vi "Meas Batch Proc QWTB Panel.vi"(8 "error in":errorcluster, 11 "session in":T1={"adc"={"niScope"={"channel cfg"=[], "sessions"=[], "multi cards"=FALSE, "channels"=0, "type"=enum."n/a", "memory [B/chn]"=0, "ext. clock [Hz]"=0.0, "samples count"=0, "use streaming"=FALSE, "proc setup"={"packet size [smpl]"=0, "current timeout [s]"=0.0, "blk2blk timeout [s]"=0.0, "event time"=timestamp(0 s since 1904-01-01), "temp sampl T [s]"=0.0, "data queue"=refnum, "stop notifier"=refnum, "proc ref"=refnum}, "sample width [B]"=0, "ranges [V]"=[], "trigger setup"={"coupling"=1, "level [V]"=0.0, "slope"=0, "mode"=enum."Immediate"}, "fs [Hz]"=0.0, "bitres [bit]"=0}, "3458A"={"channels"=[], "sync unit"={"VISA"="", "type"=enum."Picotest U6200A"}, "awg unit"={"type"=enum."Agilent 331xxA to 332xxA", "VISA"="", "enable 10MHz ref"=FALSE}, "sync mode"=enum."MASTER-SLAVE, MASTER clocked by TIMER", "streaming mode"=FALSE, "idn mode"=enum."Auto", "sampling mode"=enum."DCV", "Ts [s]"=0.0, "sample memory [B]"=0, "proc setup"={"channel id"=0, "packet size [smpl]"=0, "current timeout [s]"=0.0, "blk2blk timeout [s]"=0.0, "event time"=timestamp(0 s since 1904-01-01), "stop notifier"=refnum, "data queues"=[], "proc refs"=[], "bus semaphore"=refnum}, "sample size [B]"=0, "sample count"=0, "aux data"={"channel id"=0, "valid?"=[], "gain [V]"=[], "timestamp [s]"=[], "Ts [s]"=0.0, "abs timestamp"=timestamp(0 s since 1904-01-01), "t [deg C]"=[]}, "ranges [V]"=[], "aperture [s]"=0.0, "LEVEL trigger"={"edge"=enum."POS", "level [V]"=0.0, "coupling"=enum."DC"}, "trigger mode"=enum."AUTO", "measure temp.?"=FALSE, "disp mesages"=[], "shared bus?"=FALSE, "disable display?"=FALSE, "aper mode"=enum."Manual", "aper rules"=[]}, "dsdll"={"dsdll"={"dsdll path"=path "", "dsdll handle"=[], "output devices"=[], "capture devices"=[]}, "channels"=0, "device id"=0, "channel idns"=[], "proc setup"={"packet size [smpl]"=0, "current timeout [s]"=0.0, "blk2blk timeout [s]"=0.0, "event time"=timestamp(0 s since 1904-01-01), "data queue"=refnum, "stop notifier"=refnum, "proc ref"=refnum}, "samples count"=0, "fs [Hz]"=0.0}, "type"=enum."niScope", "channel idn str"=[], "aux instr idn str"=[], "modified?"=FALSE, "simadc"={"channels"=[], "range [V]"=0.0, "Ts step [s]"=0.0, "time [s]"=0.0, "fs [Hz]"=0.0, "count"=0, "smpl offset"=0, "set count"=0, "bit res"=0}, "force rst?"=FALSE, "exit mode"=enum."Immediate reset", "exit dly"=0.0, "exit tmr"=timestamp(0 s since 1904-01-01), "busy?"=FALSE, "accessed?"=FALSE, "QuADC session"={"channel cfg"=[], "sessions"=[], "multi cards"=FALSE, "channels"=0, "type"=enum."n/a", "memory [B/chn]"=0, "ext. clock [Hz]"=0.0, "samples count"=0, "use streaming"=FALSE, "proc setup"={"packet size [smpl]"=0, "current timeout [s]"=0.0, "blk2blk timeout [s]"=0.0, "event time"=timestamp(0 s since 1904-01-01), "temp sampl T [s]"=0.0, "data queue"=refnum, "stop notifier"=refnum, "proc ref"=refnum}, "sample width [B]"=0, "ranges [V]"=[], "trigger setup"={"coupling"=1, "level [V]"=0.0, "slope"=0, "mode"=enum."Immediate"}, "fs [Hz]"=0.0, "bitres [bit]"=0}}, "sequence"=[], "sequence setup"={"group setups"=[], "average cycles"=0, "range mode"=enum."Keep defaults", "fs mode"=enum."Frequency", "rng even"=0.0, "rng odd"=0.0, "folder"=path "", "name base"="", "meas id"=0, "settle [s]"=0.0}, "golpi"=refnum, "processing setup"={"mode"=enum."Raw", "call after avgs?"=FALSE, "calculate?"=FALSE, "raw mode"={"command"="", "result mode"=enum."Display console output (only Octave)", "res variable"=""}, "QWTB"={"QWTB path"=path "", "alg filter path"="", "alg ids"=[], "alg parameters"=[], "parsed parameters"=[], "selected alg id"="", "selected unc mode"=enum."None", "qwtb mcc"=100, "qwtb timeout"=90, "qwtb covg"=95.0, "qwtb ofs"=0, "qwtb lim data"=0, "multicore"={"jobs folder"=path "", "cores"=0, "max jobs"=0, "mode"=enum."Singlecore"}, "unc once?"=FALSE}}, "corrections"={"transducers"={"channels"=[], "last path"=path ""}, "digitizer"={"last path"=path "", "channel paths"=[], "channel idns"=[], "correction name"="", "channel names"=[], "folders to copy"=[], "channel valid"=[], "correction path"=path "", "correction rel path"="", "rel folders to copy"=[]}}, "assist cfg"={"P"=0, "Q"=0, "rel shift"=0.0, "ref freq"=0.0, "min fs"=0.0, "max fs tol"=0.0, "min int"=0.0, "max int"=0.0, "max err"=0.0, "max timeout"=0.0}} {"corrections"."transducers"."channels"."Phase index" min=1 step=1; "adc"."QuADC session"."trigger setup"."level [V]" format="%.2f"; "adc"."QuADC session"."trigger setup"."coupling" items=["AC"=0, "DC"=1, "HF Reject"=3, "LF Reject"=4, "AC Plus HF Reject"=1001]; "adc"."QuADC session"."channel cfg"."Clock fr. (Hz)" min=0.0 format="%#_9p"; "adc"."QuADC session"."channel cfg"."Number of JJ" min=1; "adc"."QuADC session"."channel cfg"."Range [Vpk]" min=0.0; "adc"."QuADC session"."channel cfg"."Channel" min=0; "adc"."3458A"."channels"."Range [Vpk]" min=0.0; "adc"."niScope"."trigger setup"."level [V]" format="%.2f"; "adc"."niScope"."trigger setup"."coupling" items=["AC"=0, "DC"=1, "HF Reject"=3, "LF Reject"=4, "AC Plus HF Reject"=1001]; "adc"."niScope"."channel cfg"."Range [Vpk]" min=0.0; "adc"."niScope"."channel cfg"."Channel" min=0}) -> (0 "error out":errorcluster, 3 "session out":T1={"adc"={"niScope"={"channel cfg"=[], "sessions"=[], "multi cards"=FALSE, "channels"=0, "type"=enum."n/a", "memory [B/chn]"=0, "ext. clock [Hz]"=0.0, "samples count"=0, "use streaming"=FALSE, "proc setup"={"packet size [smpl]"=0, "current timeout [s]"=0.0, "blk2blk timeout [s]"=0.0, "event time"=timestamp(0 s since 1904-01-01), "temp sampl T [s]"=0.0, "data queue"=refnum, "stop notifier"=refnum, "proc ref"=refnum}, "sample width [B]"=0, "ranges [V]"=[], "trigger setup"={"coupling"=1, "level [V]"=0.0, "slope"=0, "mode"=enum."Immediate"}, "fs [Hz]"=0.0, "bitres [bit]"=0}, "3458A"={"channels"=[], "sync unit"={"VISA"="", "type"=enum."Picotest U6200A"}, "awg unit"={"type"=enum."Agilent 331xxA to 332xxA", "VISA"="", "enable 10MHz ref"=FALSE}, "sync mode"=enum."MASTER-SLAVE, MASTER clocked by TIMER", "streaming mode"=FALSE, "idn mode"=enum."Auto", "sampling mode"=enum."DCV", "Ts [s]"=0.0, "sample memory [B]"=0, "proc setup"={"channel id"=0, "packet size [smpl]"=0, "current timeout [s]"=0.0, "blk2blk timeout [s]"=0.0, "event time"=timestamp(0 s since 1904-01-01), "stop notifier"=refnum, "data queues"=[], "proc refs"=[], "bus semaphore"=refnum}, "sample size [B]"=0, "sample count"=0, "aux data"={"channel id"=0, "valid?"=[], "gain [V]"=[], "timestamp [s]"=[], "Ts [s]"=0.0, "abs timestamp"=timestamp(0 s since 1904-01-01), "t [deg C]"=[]}, "ranges [V]"=[], "aperture [s]"=0.0, "LEVEL trigger"={"edge"=enum."POS", "level [V]"=0.0, "coupling"=enum."DC"}, "trigger mode"=enum."AUTO", "measure temp.?"=FALSE, "disp mesages"=[], "shared bus?"=FALSE, "disable display?"=FALSE, "aper mode"=enum."Manual", "aper rules"=[]}, "dsdll"={"dsdll"={"dsdll path"=path "", "dsdll handle"=[], "output devices"=[], "capture devices"=[]}, "channels"=0, "device id"=0, "channel idns"=[], "proc setup"={"packet size [smpl]"=0, "current timeout [s]"=0.0, "blk2blk timeout [s]"=0.0, "event time"=timestamp(0 s since 1904-01-01), "data queue"=refnum, "stop notifier"=refnum, "proc ref"=refnum}, "samples count"=0, "fs [Hz]"=0.0}, "type"=enum."niScope", "channel idn str"=[], "aux instr idn str"=[], "modified?"=FALSE, "simadc"={"channels"=[], "range [V]"=0.0, "Ts step [s]"=0.0, "time [s]"=0.0, "fs [Hz]"=0.0, "count"=0, "smpl offset"=0, "set count"=0, "bit res"=0}, "force rst?"=FALSE, "exit mode"=enum."Immediate reset", "exit dly"=0.0, "exit tmr"=timestamp(0 s since 1904-01-01), "busy?"=FALSE, "accessed?"=FALSE, "QuADC session"={"channel cfg"=[], "sessions"=[], "multi cards"=FALSE, "channels"=0, "type"=enum."n/a", "memory [B/chn]"=0, "ext. clock [Hz]"=0.0, "samples count"=0, "use streaming"=FALSE, "proc setup"={"packet size [smpl]"=0, "current timeout [s]"=0.0, "blk2blk timeout [s]"=0.0, "event time"=timestamp(0 s since 1904-01-01), "temp sampl T [s]"=0.0, "data queue"=refnum, "stop notifier"=refnum, "proc ref"=refnum}, "sample width [B]"=0, "ranges [V]"=[], "trigger setup"={"coupling"=1, "level [V]"=0.0, "slope"=0, "mode"=enum."Immediate"}, "fs [Hz]"=0.0, "bitres [bit]"=0}}, "sequence"=[], "sequence setup"={"group setups"=[], "average cycles"=0, "range mode"=enum."Keep defaults", "fs mode"=enum."Frequency", "rng even"=0.0, "rng odd"=0.0, "folder"=path "", "name base"="", "meas id"=0, "settle [s]"=0.0}, "golpi"=refnum, "processing setup"={"mode"=enum."Raw", "call after avgs?"=FALSE, "calculate?"=FALSE, "raw mode"={"command"="", "result mode"=enum."Display console output (only Octave)", "res variable"=""}, "QWTB"={"QWTB path"=path "", "alg filter path"="", "alg ids"=[], "alg parameters"=[], "parsed parameters"=[], "selected alg id"="", "selected unc mode"=enum."None", "qwtb mcc"=100, "qwtb timeout"=90, "qwtb covg"=95.0, "qwtb ofs"=0, "qwtb lim data"=0, "multicore"={"jobs folder"=path "", "cores"=0, "max jobs"=0, "mode"=enum."Singlecore"}, "unc once?"=FALSE}}, "corrections"={"transducers"={"channels"=[], "last path"=path ""}, "digitizer"={"last path"=path "", "channel paths"=[], "channel idns"=[], "correction name"="", "channel names"=[], "folders to copy"=[], "channel valid"=[], "correction path"=path "", "correction rel path"="", "rel folders to copy"=[]}}, "assist cfg"={"P"=0, "Q"=0, "rel shift"=0.0, "ref freq"=0.0, "min fs"=0.0, "max fs tol"=0.0, "min int"=0.0, "max int"=0.0, "max err"=0.0, "max timeout"=0.0}} {"corrections"."transducers"."channels"."Phase index" min=1 step=1; "adc"."QuADC session"."trigger setup"."level [V]" format="%.2f"; "adc"."QuADC session"."trigger setup"."coupling" items=["AC"=0, "DC"=1, "HF Reject"=3, "LF Reject"=4, "AC Plus HF Reject"=1001]; "adc"."QuADC session"."channel cfg"."Clock fr. (Hz)" min=0.0 format="%#_9p"; "adc"."QuADC session"."channel cfg"."Number of JJ" min=1; "adc"."QuADC session"."channel cfg"."Range [Vpk]" min=0.0; "adc"."QuADC session"."channel cfg"."Channel" min=0; "adc"."3458A"."channels"."Range [Vpk]" min=0.0; "adc"."niScope"."trigger setup"."level [V]" format="%.2f"; "adc"."niScope"."trigger setup"."coupling" items=["AC"=0, "DC"=1, "HF Reject"=3, "LF Reject"=4, "AC Plus HF Reject"=1001]; "adc"."niScope"."channel cfg"."Range [Vpk]" min=0.0; "adc"."niScope"."channel cfg"."Channel" min=0})   [LabVIEW 2018]
doc: "Main panel for QWTB batch processing."
uses:
  Meas Session.ctl
  adc/ADC Session.ctl
  drivers/niScope/niScope Session.ctl
  drivers/niScope/niScope Virtual Channel Config.ctl
  drivers/niScope/niScope Virtual Channel Mode.ctl
  drivers/niScope/niScope Virtual Channel Input Z.ctl
  drivers/niScope/niScope Virtual Channel Coupling.ctl
  drivers/niScope/niScope Type.ctl
  drivers/niScope/niScope Digitizing Process Options.ctl
  drivers/niScope/niScope Data Packet.ctl
  drivers/niScope/niScope Trigger Setup.ctl
  <instrlib>/niScope/Controls/niScope trigger coupling.ctl
  <instrlib>/niScope/Controls/niScope trigger slope.ctl
  drivers/DMM/3458A Digitizer Session.ctl
  drivers/DMM/3458A Virtual Channel Config.ctl
  drivers/Counter/Counter Session.ctl
  drivers/Counter/Counter Type.ctl
  drivers/AWG/AWG Session.ctl
  drivers/AWG/AWG Type.ctl
  drivers/DMM/3458A Sync Mode.ctl
  drivers/DMM/3458A Idn Mode.ctl
  drivers/DMM/3458A Digitizing Low Levels/Configure/Sampling Mode.ctl
  drivers/DMM/3458A Digitizing Process Options.ctl
  drivers/DMM/3458A Data Packet.ctl
  drivers/DMM/3458A Aux Record Data.ctl
  drivers/DMM/3458A Digitizing Low Levels/Configure/Level Setup.ctl
  drivers/DMM/3458A Digitizing Low Levels/Configure/First Sample Trigger.ctl
  drivers/DMM/3458A Aperture Selection Mode.ctl
  drivers/dsdll/DSDLL Session.ctl
  drivers/dsdll/dsdll source distribution/dsdll_instance.ctl
  drivers/dsdll/dsdll source distribution/dsdll_device_record.ctl
  drivers/dsdll/DSDLL Process Config.ctl
  drivers/dsdll/DSDLL Data Packet.ctl
  adc/ADC Type.ctl
  drivers/simulated_adc/SimAdc Config.ctl
  drivers/simulated_adc/SimAdc Channel Cfg.ctl
  adc/ADC On Close Action.ctl
  drivers/Quatsch_driver/QuADCDriver/QuADC Session.ctl
  drivers/Quatsch_driver/QuADCDriver/QuADC Virtual Channel Config.ctl
  drivers/Quatsch_driver/QuADCDriver/QuADC Virtual Channel Mode.ctl
  drivers/Quatsch_driver/QuADCDriver/QuADC Virtual Channel Input Z.ctl
  drivers/Quatsch_driver/QuADCDriver/QuADC Virtual Channel Coupling.ctl
  drivers/Quatsch_driver/QuADCDriver/QuADC Type.ctl
  drivers/Quatsch_driver/QuADCDriver/QuADC Digitizing Process Options.ctl
  drivers/Quatsch_driver/QuADCDriver/QuADC Data Packet.ctl
  drivers/Quatsch_driver/QuADCDriver/QuADC Trigger Setup.ctl
  Meas Sequence Item.ctl
  Meas Sampling Configuration.ctl
  adc/ADC Trig Config.ctl
  adc/ADC Trig Mode Source.ctl
  adc/ADC Trig Coupling.ctl
  adc/ADC Trig Slope.ctl
  Meas Proc QWTB Algorithm Parameter Data.ctl
  Meas Sequence Configuration.ctl
  Meas Range Mode.ctl
  Meas Sampling Rate Mode.ctl
  octave/golpi/mpc/golpi_session_ref.ctl
  octave/golpi/mpc/golpi_session.ctl
  octave/golpi/GOLPI Library.lvlibp/Public/GOLPI reference Type Def.ctl
  octave/golpi/GOLPI Library.lvlibp/LV Process source distribution/Pipe Handle.ctl
  Meas Process Config.ctl
  Meas Process Mode.ctl
  Meas Process Raw Config.ctl
  Meas Process Raw Result Mode.ctl
  Meas Proc QWTB Setup.ctl
  Meas Proc QWTB Uncertainty Mode.ctl
  Meas Proc QWTB Multicore Setup.ctl
  Meas Proc QWTB Multicore Type.ctl
  Corrections/Corr Setup.ctl
  Corrections/Corr Tranducer Item.ctl
  Corrections/Corr Digitizers.ctl
  Assist/Assist Panel Setup.ctl
  varilib/SGUI Assign References Mode.ctl
  octave/infolib.lvlibp/Private/Get key polymorph parts/GetI64.vi
  octave/infolib.lvlibp/Private/Get matrix polymorph parts/Get 1D String.vi
  <vilib>/Utility/error.llb/Error Cluster From Error Code.vi
  varilib/SGUI Assign Multiple Strings With Tags By Label.vi
  <vilib>/ErrorRing/Error Ring.xnode
  octave/infolib.lvlibp
  varilib/varilib.lvlib
  drivers/niScope/niScope Virtual Digitizer.lvlib
  drivers/DMM/3458A Virtual Digitizer.lvlib
  drivers/Counter/Counter.lvlib
  drivers/AWG/AWG.lvlib
  drivers/DMM/3458A Digitizing Low Levels/3458A Digitizing Low Levels.lvlib
  drivers/dsdll/DSDLL Virtual Digitizer.lvlib
  octave/golpi/GOLPI Library.lvlibp/LV Process source distribution/LV Process library.lvlib
  octave/golpi/GOLPI Library.lvlibp
  octave/golpi/mpc/GOLPI Multi Process.lvlib
  drivers/Quatsch_driver/QuADCDriver/QuADC Virtual Digitizer.lvlib
  drivers/dsdll/dsdll source distribution/dsdll.lvlib
panel:
  in  "path history":path caption="Select measurement session"
  in  "btn stop":bool
  out "rec ids":i32[](array[numeric])
  out "group ids unique":i32[](array[numeric])
  out "status":string caption="Status"
  out "group ids":i32[](array[numeric])
  in  "rec list":i32[](listbox) caption="Records available"
  in  "btn cancel":bool
  in  "btn ok":bool
  in  "grp list":i32[](listbox) caption="Groups available"
  in  "meas path":path caption="Select measurement session"
  in  "btn proc":bool
  # "ADC:"
  # "IP Address"
  # "."
  # "."
  # "."
  # ":"
  # "ADC:"
  # "IP Address"
  # "."
  # "."
  # "."
  # ":"
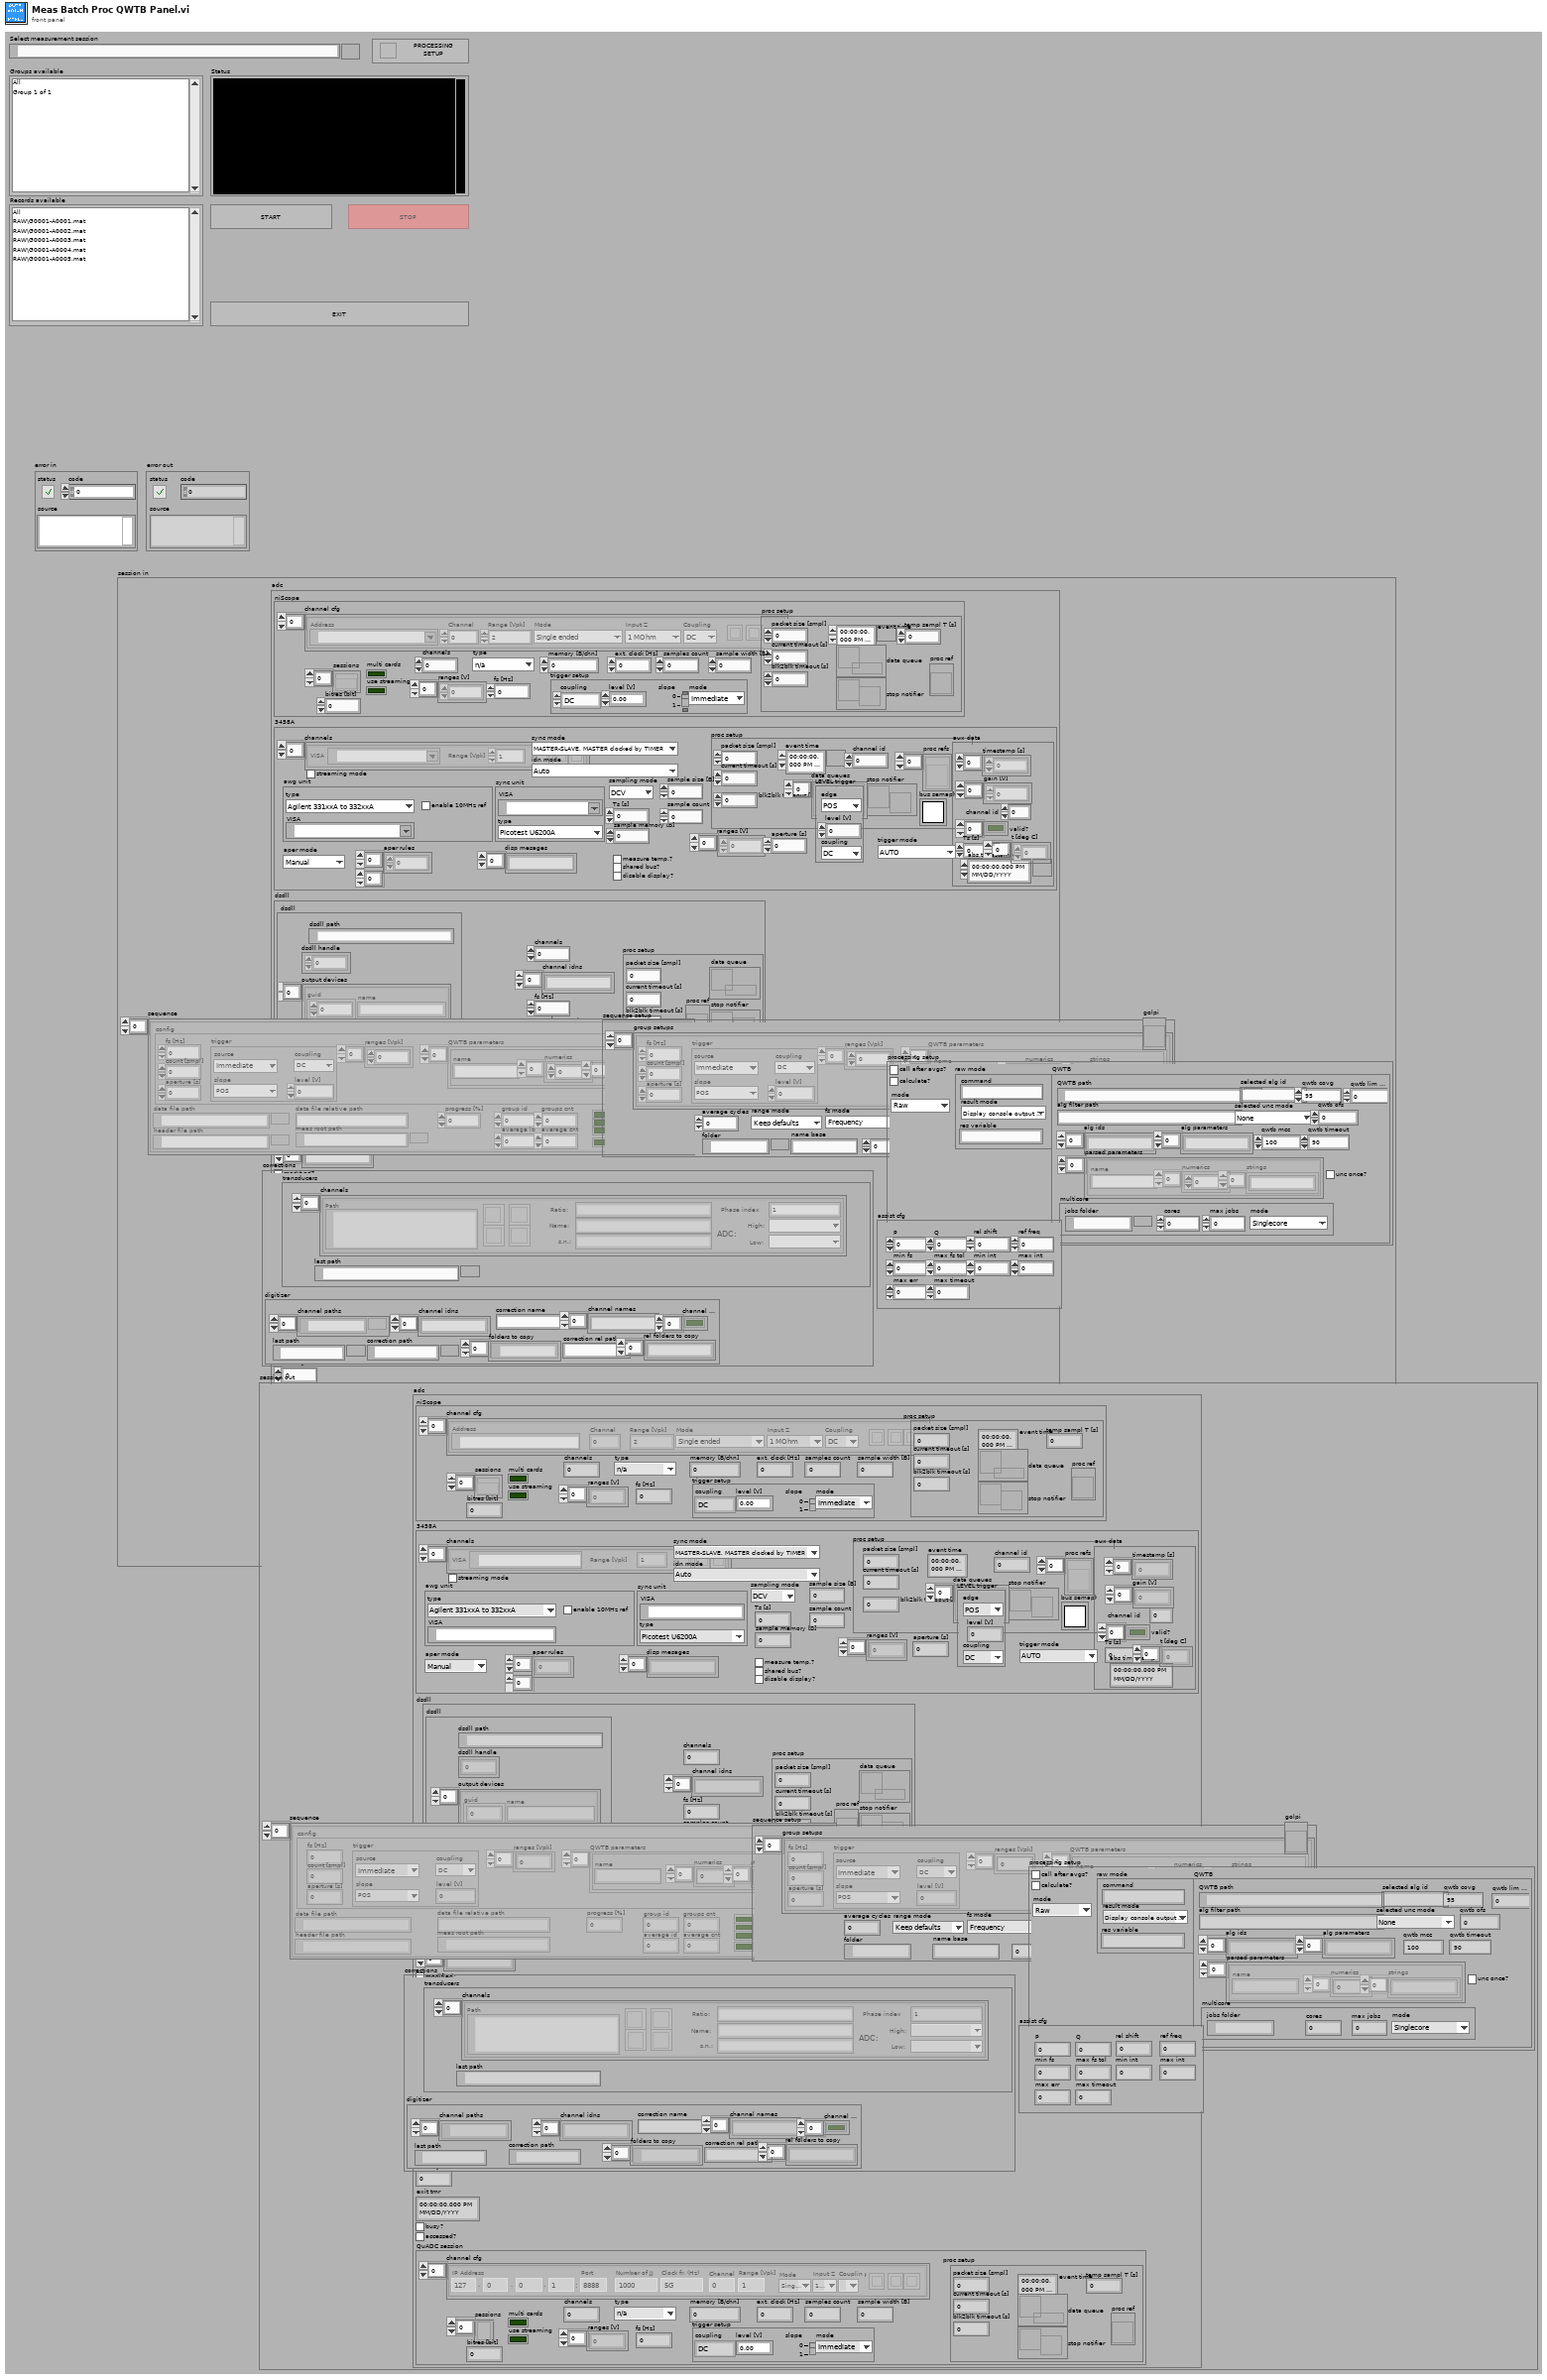
[diagram p1: front panel]
types:
  T1 = typedef "Meas Session.ctl" = cluster{"adc":T2, "sequence":T44[], "sequence setup":T51, "golpi":T54, "processing setup":T55, "corrections":T63, "assist cfg":T66}
  T2 = typedef "ADC Session.ctl" = cluster{"niScope":T3, "3458A":T13, "dsdll":T28, "type":T32, "channel idn str":string[], "aux instr idn str":string[], "modified?":bool, "simadc":T33, "force rst?":bool, "exit mode":T35, "exit dly":dbl, "exit tmr":timestamp, "busy?":bool, "accessed?":bool, "QuADC session":T36}
  T3 = typedef "niScope Virtual Digitizer.lvlib/niScope Session.ctl" = cluster{"channel cfg":T4[], "sessions":refnum<k20>[], "multi cards":bool, "channels":i32, "type":T8, "memory [B/chn]":i32, "ext. clock [Hz]":dbl, "samples count":i64, "use streaming":bool, "proc setup":T9, "sample width [B]":i32, "ranges [V]":dbl[], "trigger setup":T10, "fs [Hz]":dbl, "bitres [bit]":i32}
  T4 = typedef "niScope Virtual Digitizer.lvlib/niScope Virtual Channel Config.ctl" = cluster{"Address":refnum<k15>, "Channel":i32, "Mode":T5, "Input Z":T6, "Coupling":T7, "Range [Vpk]":dbl, "btn clr":bool, "btn up":bool, "btn down":bool}
  T5 = typedef "niScope Virtual Digitizer.lvlib/niScope Virtual Channel Mode.ctl" = enum16{"Single ended", "Unbal. differential", "Differential"}
  T6 = typedef "niScope Virtual Digitizer.lvlib/niScope Virtual Channel Input Z.ctl" = enum16{"1 MOhm", "50 Ohm"}
  T7 = typedef "niScope Virtual Digitizer.lvlib/niScope Virtual Channel Coupling.ctl" = enum16{"AC", "DC", "GND"}
  T8 = typedef "niScope Virtual Digitizer.lvlib/niScope Type.ctl" = enum16{"n/a", "5922"}
  T9 = typedef "niScope Virtual Digitizer.lvlib/niScope Digitizing Process Options.ctl" = cluster{"packet size [smpl]":i64, "current timeout [s]":dbl, "blk2blk timeout [s]":dbl, "event time":timestamp, "temp sampl T [s]":dbl, "data queue":refnum<queue>, "stop notifier":refnum<notifier>, "proc ref":refnum<vi>}
  T10 = typedef "niScope Virtual Digitizer.lvlib/niScope Trigger Setup.ctl" = cluster{"coupling":T11, "level [V]":dbl, "slope":T12, "mode":enum16{"Immediate", "External", "Level"}}
  T11 = typedef "niScope trigger coupling.ctl" = u16
  T12 = typedef "niScope trigger slope.ctl" = i32
  T13 = typedef "3458A Virtual Digitizer.lvlib/3458A Digitizer Session.ctl" = cluster{"channels":T14[], "sync unit":T15, "awg unit":T17, "sync mode":T19, "streaming mode":bool, "idn mode":T20, "sampling mode":T21, "Ts [s]":dbl, "sample memory [B]":i32, "proc setup":T22, "sample size [B]":i32, "sample count":i32, "aux data":T24, "ranges [V]":dbl[], "aperture [s]":dbl, "LEVEL trigger":T25, "trigger mode":T26, "measure temp.?":bool, "disp mesages":string[], "shared bus?":bool, "disable display?":bool, "aper mode":T27, "aper rules":dbl[][]}
  T14 = typedef "3458A Virtual Digitizer.lvlib/3458A Virtual Channel Config.ctl" = cluster{"VISA":refnum<visa-resource-name>, "Range [Vpk]":dbl, "btn clr":bool, "btn up":bool, "btn down":bool}
  T15 = typedef "Counter.lvlib/Counter Session.ctl" = cluster{"VISA":refnum<visa-resource-name>, "type":T16}
  T16 = typedef "Counter.lvlib/Counter Type.ctl" = enum16{"Picotest U6200A", "dummy"}
  T17 = typedef "AWG.lvlib/AWG Session.ctl" = cluster{"type":T18, "VISA":refnum<visa-resource-name>, "enable 10MHz ref":bool}
  T18 = typedef "AWG.lvlib/AWG Type.ctl" = enum16{"Agilent 331xxA to 332xxA", "Agilent 335xxA to 336xxA", "Tektronix AFG3101C", "dummy"}
  T19 = typedef "3458A Virtual Digitizer.lvlib/3458A Sync Mode.ctl" = enum16{"MASTER-SLAVE, MASTER clocked by TIMER", "MASTER-SLAVE, MASTER clocked by AWG", "ALL clocked by AWG", "MASTER-SLAVE, ALL clocked by TIMER", "ALL clocked by AWG with DFLL"}
  T20 = typedef "3458A Virtual Digitizer.lvlib/3458A Idn Mode.ctl" = enum16{"Auto", "Sequential (chn A, chn B, ...)", "From calibration string"}
  T21 = typedef "3458A Virtual Digitizer.lvlib/3458A Digitizing Low Levels.lvlib/Sampling Mode.ctl" = enum16{"DCV", "DSDC", "DSAC"}
  T22 = typedef "3458A Virtual Digitizer.lvlib/3458A Digitizing Process Options.ctl" = cluster{"channel id":i32, "packet size [smpl]":i32, "current timeout [s]":dbl, "blk2blk timeout [s]":dbl, "event time":timestamp, "stop notifier":refnum<notifier>, "data queues":refnum<queue>[], "proc refs":refnum<vi>[], "bus semaphore":T23}
  T23 = typedef "Semaphore RefNum" = refnum<k1>
  T24 = typedef "3458A Virtual Digitizer.lvlib/3458A Aux Record Data.ctl" = cluster{"channel id":i32, "valid?":bool[], "gain [V]":dbl[], "timestamp [s]":dbl[], "Ts [s]":dbl, "abs timestamp":timestamp, "t [deg C]":dbl[]}
  T25 = typedef "3458A Virtual Digitizer.lvlib/3458A Digitizing Low Levels.lvlib/Level Setup.ctl" = cluster{"edge":enum16{"POS", "NEG"}, "level [V]":dbl, "coupling":enum16{"DC", "AC"}}
  T26 = typedef "3458A Virtual Digitizer.lvlib/3458A Digitizing Low Levels.lvlib/First Sample Trigger.ctl" = enum16{"AUTO", "EXT", "SYN", "SGL", "HOLD", "LEVEL"}
  T27 = typedef "3458A Virtual Digitizer.lvlib/3458A Aperture Selection Mode.ctl" = enum16{"Manual", "Maximum", "Table"}
  T28 = typedef "DSDLL Virtual Digitizer.lvlib/DSDLL Session.ctl" = cluster{"dsdll":T29, "channels":i32, "device id":i32, "channel idns":string[], "proc setup":T31, "samples count":i32, "fs [Hz]":dbl}
  T29 = typedef "dsdll.lvlib/dsdll_instance.ctl" = cluster{"dsdll path":path, "dsdll handle":u8[], "output devices":T30[], "capture devices":T30[]}
  T30 = typedef "dsdll.lvlib/dsdll_device_record.ctl" = cluster{"guid":u8[], "name":string}
  T31 = typedef "DSDLL Virtual Digitizer.lvlib/DSDLL Process Config.ctl" = cluster{"packet size [smpl]":i32, "current timeout [s]":dbl, "blk2blk timeout [s]":dbl, "event time":timestamp, "data queue":refnum<queue>, "stop notifier":refnum<notifier>, "proc ref":refnum<vi>}
  T32 = typedef "ADC Type.ctl" = enum16{"niScope", "3458A", "DirectSound DLL", "dummy", "QuADC"}
  T33 = typedef "SimAdc Config.ctl" = cluster{"channels":T34[], "range [V]":dbl, "Ts step [s]":dbl, "time [s]":dbl, "fs [Hz]":dbl, "count":i64, "smpl offset":i64, "set count":i64, "bit res":i32}
  T34 = typedef "SimAdc Channel Cfg.ctl" = cluster{"harmonics":dbl[][], "btn clear":bool, "noise":dbl, "fundamental [Hz]":dbl}
  T35 = typedef "ADC On Close Action.ctl" = enum16{"Immediate reset", "Delayed reset"}
  T36 = typedef "QuADC Virtual Digitizer.lvlib/QuADC Session.ctl" = cluster{"channel cfg":T37[], "sessions":refnum<k5>[], "multi cards":bool, "channels":i32, "type":T41, "memory [B/chn]":i32, "ext. clock [Hz]":dbl, "samples count":i64, "use streaming":bool, "proc setup":T42, "sample width [B]":i32, "ranges [V]":dbl[], "trigger setup":T43, "fs [Hz]":dbl, "bitres [bit]":i32}
  T37 = typedef "QuADC Virtual Digitizer.lvlib/QuADC Virtual Channel Config.ctl" = cluster{"Channel":i32, "Mode":T38, "Input Z":T39, "Coupling":T40, "Range [Vpk]":dbl, "btn clr":bool, "btn up":bool, "btn down":bool, "IP address A":u8, "IP address B":u8, "IP address C":u8, "IP address D":u8, "Port":u16, "Number of JJ":u32, "Clock fr. (Hz)":dbl}
  T38 = typedef "QuADC Virtual Digitizer.lvlib/QuADC Virtual Channel Mode.ctl" = enum16{"Single ended", "Unbal. differential", "Differential"}
  T39 = typedef "QuADC Virtual Digitizer.lvlib/QuADC Virtual Channel Input Z.ctl" = enum16{"1 MOhm", "50 Ohm"}
  T40 = typedef "QuADC Virtual Digitizer.lvlib/QuADC Virtual Channel Coupling.ctl" = enum16{"AC", "DC", "GND"}
  T41 = typedef "QuADC Virtual Digitizer.lvlib/QuADC Type.ctl" = enum16{"n/a", "v1"}
  T42 = typedef "QuADC Virtual Digitizer.lvlib/QuADC Digitizing Process Options.ctl" = cluster{"packet size [smpl]":i64, "current timeout [s]":dbl, "blk2blk timeout [s]":dbl, "event time":timestamp, "temp sampl T [s]":dbl, "data queue":refnum<queue>, "stop notifier":refnum<notifier>, "proc ref":refnum<vi>}
  T43 = typedef "QuADC Virtual Digitizer.lvlib/QuADC Trigger Setup.ctl" = cluster{"coupling":T11, "level [V]":dbl, "slope":T12, "mode":enum16{"Immediate", "External", "Level"}}
  T44 = typedef "Meas Sequence Item.ctl" = cluster{"config":T45, "data file path":path, "header file path":path, "group id":i32, "average id":i32, "group done?":bool, "adc modified?":bool, "source modified?":bool, "progress [%]":dbl, "groups cnt":i32, "average cnt":i32, "data file relative path":string, "meas root path":path, "calculate?":bool}
  T45 = typedef "Meas Sampling Configuration.ctl" = cluster{"fs [Hz]":dbl, "count [smpl]":i64, "aperture [s]":dbl, "trigger":T46, "ranges [Vpk]":dbl[], "QWTB parameters":T50[]}
  T46 = typedef "ADC Trig Config.ctl" = cluster{"source":T47, "level [V]":dbl, "coupling":T48, "slope":T49}
  T47 = typedef "ADC Trig Mode Source.ctl" = enum16{"Immediate", "External", "Level"}
  T48 = typedef "ADC Trig Coupling.ctl" = enum16{"DC", "AC"}
  T49 = typedef "ADC Trig Slope.ctl" = enum16{"POS", "NEG"}
  T50 = typedef "Meas Proc QWTB Algorithm Parameter Data.ctl" = cluster{"name":string, "numerics":dbl[], "strings":string[]}
  T51 = typedef "Meas Sequence Configuration.ctl" = cluster{"group setups":T45[], "average cycles":i32, "range mode":T52, "fs mode":T53, "rng even":dbl, "rng odd":dbl, "folder":path, "name base":string, "meas id":i32, "settle [s]":dbl}
  T52 = typedef "Meas Range Mode.ctl" = enum16{"Keep defaults", "Set All channels", "Set Odd and Even channels"}
  T53 = typedef "Meas Sampling Rate Mode.ctl" = enum16{"Frequency", "Period"}
  T54 = typedef "GOLPI Multi Process.lvlib/golpi_session_ref.ctl" = refnum<vi>
  T55 = typedef "Meas Process Config.ctl" = cluster{"mode":T56, "call after avgs?":bool, "calculate?":bool, "raw mode":T57, "QWTB":T59}
  T56 = typedef "Meas Process Mode.ctl" = enum16{"Raw", "QWTB"}
  T57 = typedef "Meas Process Raw Config.ctl" = cluster{"command":string, "result mode":T58, "res variable":string}
  T58 = typedef "Meas Process Raw Result Mode.ctl" = enum16{"Display console output (only Octave)", "Display string variable", "Display result file %respath%"}
  T59 = typedef "Meas Proc QWTB Setup.ctl" = cluster{"QWTB path":path, "alg filter path":string, "alg ids":string[], "alg parameters":string[], "parsed parameters":T50[], "selected alg id":string, "selected unc mode":T60, "qwtb mcc":i32, "qwtb timeout":i32, "qwtb covg":dbl, "qwtb ofs":i64, "qwtb lim data":i64, "multicore":T61, "unc once?":bool}
  T60 = typedef "Meas Proc QWTB Uncertainty Mode.ctl" = enum16{"None", "GUF", "Monte Carlo"}
  T61 = typedef "Meas Proc QWTB Multicore Setup.ctl" = cluster{"jobs folder":path, "cores":i32, "max jobs":i32, "mode":T62}
  T62 = typedef "Meas Proc QWTB Multicore Type.ctl" = enum16{"Singlecore", "Multicore", "Multistation"}
  T63 = typedef "Corr Setup.ctl" = cluster{"transducers":cluster{"channels":T64[], "last path":path}, "digitizer":T65}
  T64 = typedef "Corr Tranducer Item.ctl" = cluster{"Path":path, "Ratio:":string, "Name:":string, "btn rem":bool, "btn up":bool, "btn down":bool, "s.n.:":string, "btn open":bool, "ratio o/i":dbl, "chn hi":u16, "chn lo":u16, "Phase index":i32}
  T65 = typedef "Corr Digitizers.ctl" = cluster{"last path":path, "channel paths":path[], "channel idns":string[], "correction name":string, "channel names":string[], "folders to copy":path[], "channel valid":bool[], "correction path":path, "correction rel path":string, "rel folders to copy":string[]}
  T66 = typedef "Assist Panel Setup.ctl" = cluster{"P":i32, "Q":i32, "rel shift":dbl, "ref freq":dbl, "min fs":dbl, "max fs tol":dbl, "min int":dbl, "max int":dbl, "max err":dbl, "max timeout":dbl}
  T67 = typedef "varilib.lvlib/SGUI Assign References Mode.ctl" = enum16{"Add to stack", "Overwrite", "Release last", "Release ID"}
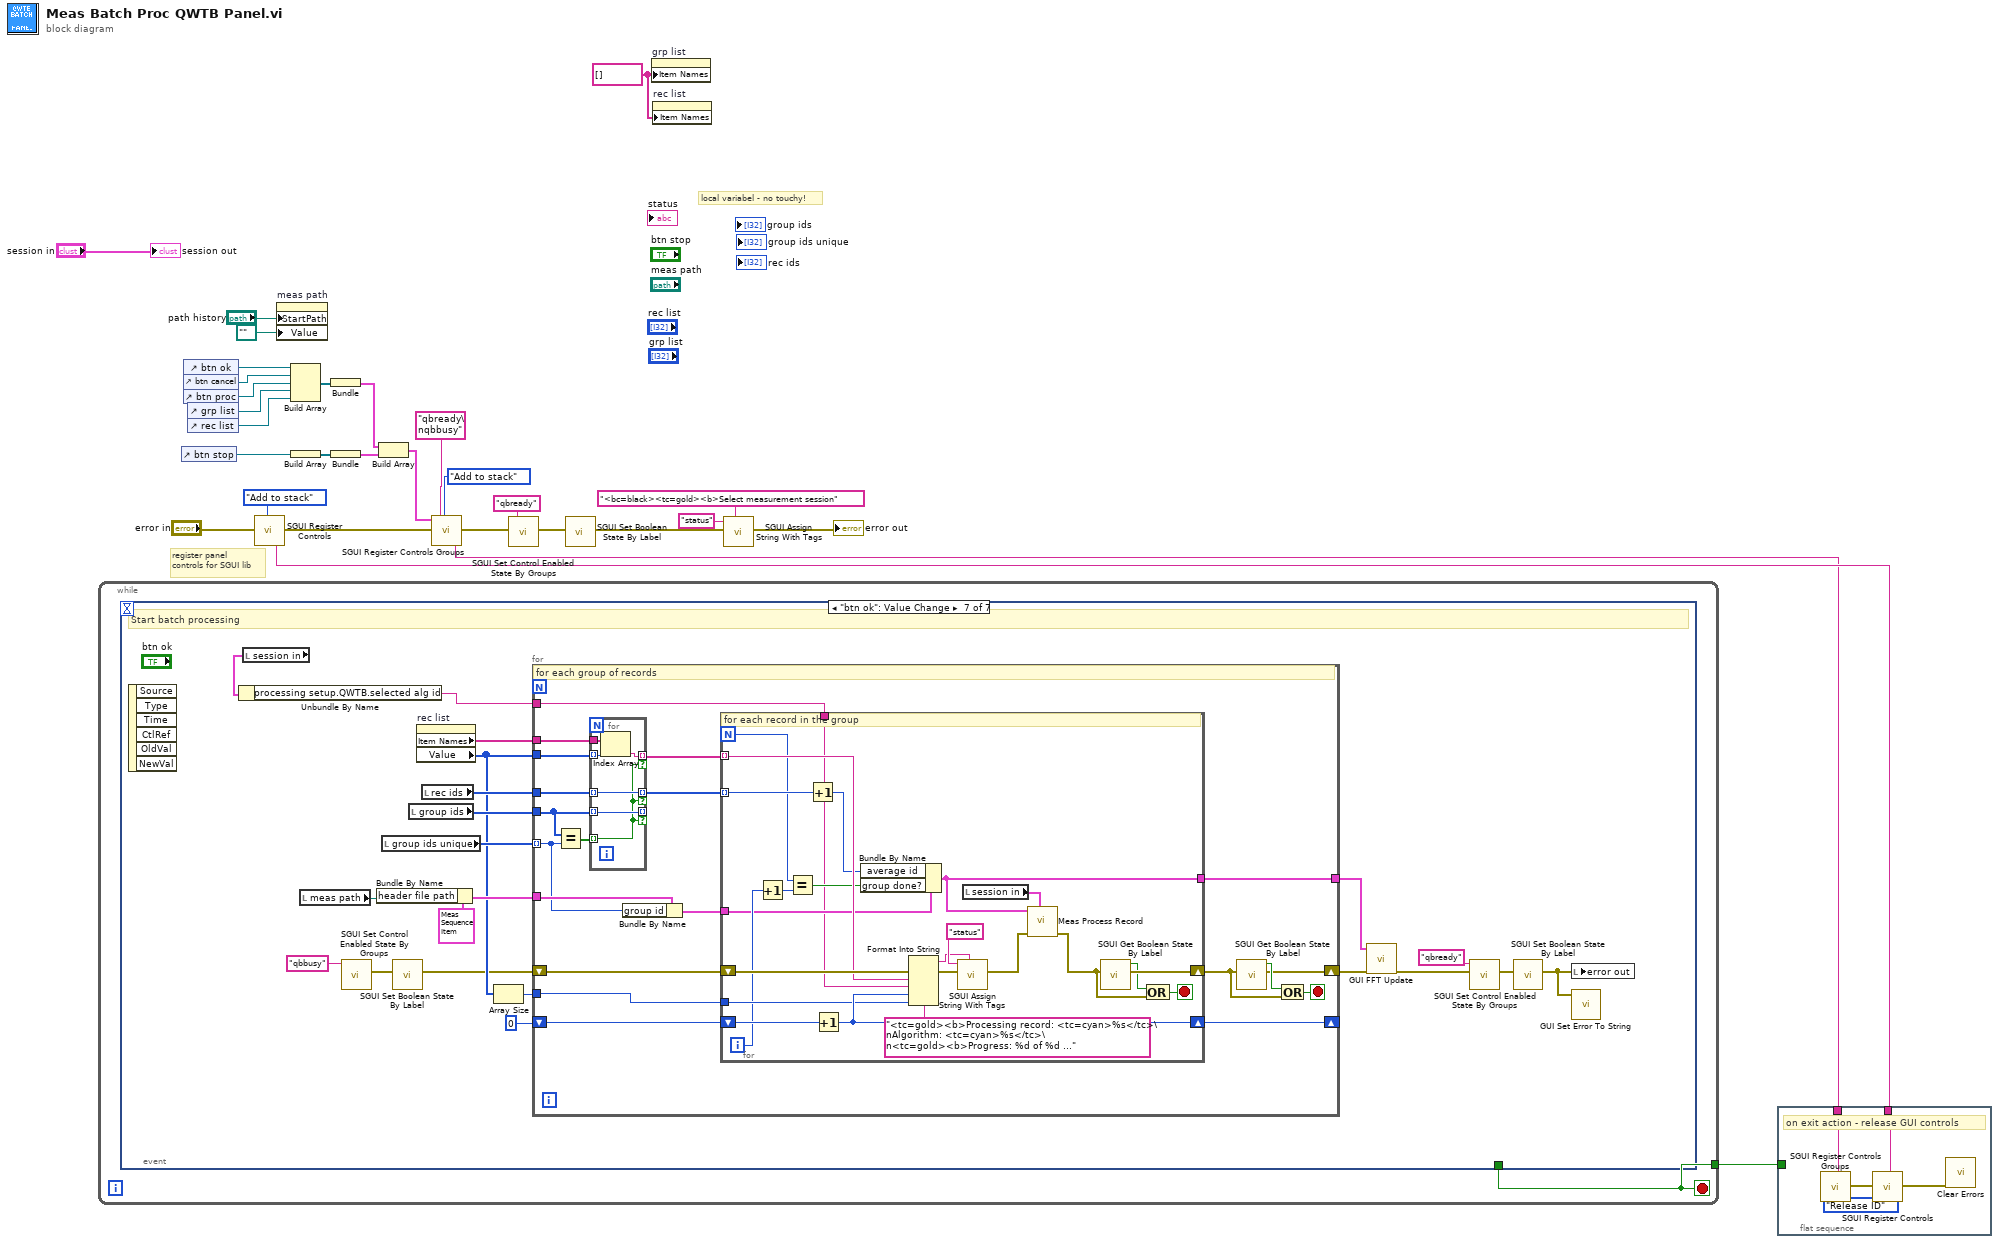
[diagram p0: block diagram]
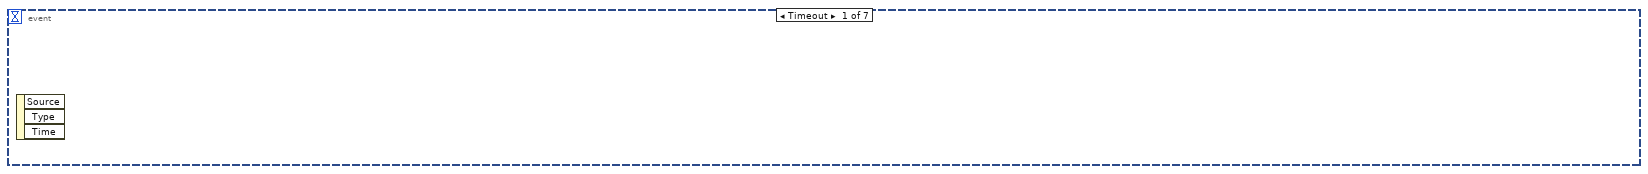
[diagram p2: hidden frame]
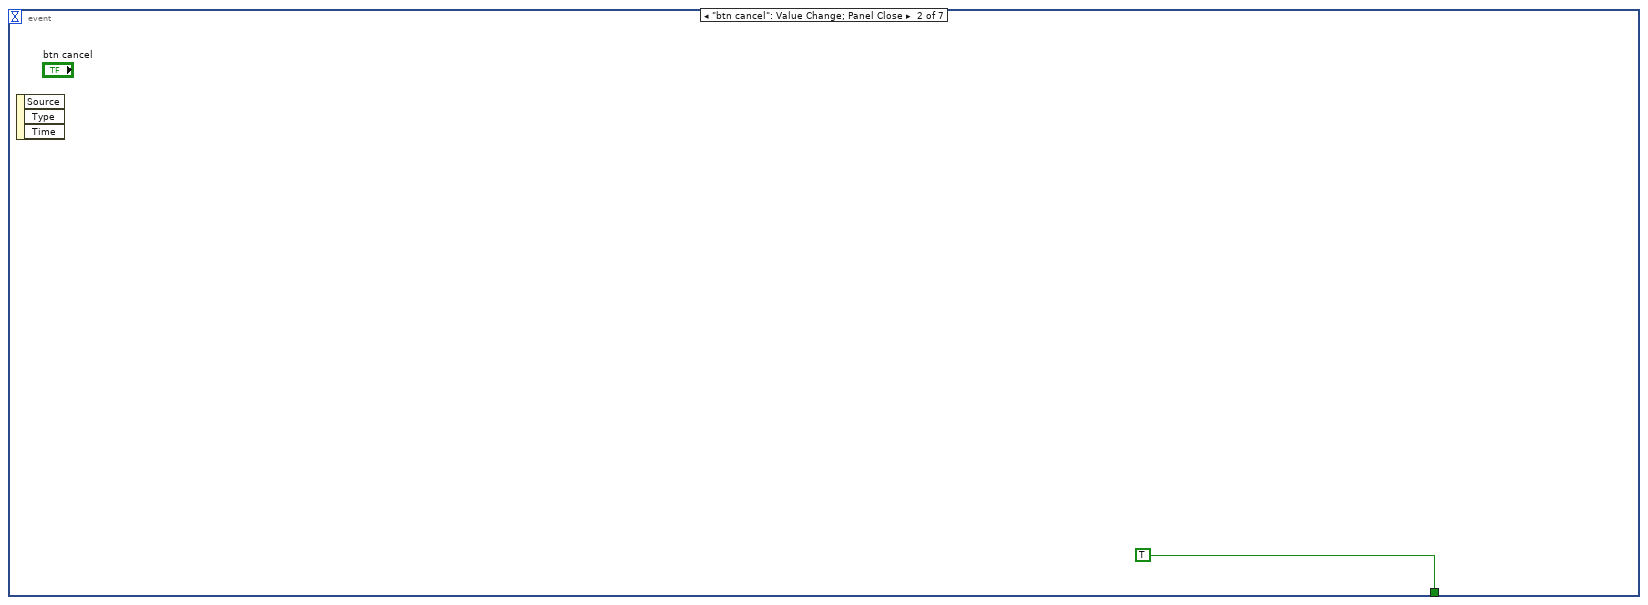
[diagram p3: hidden frame]
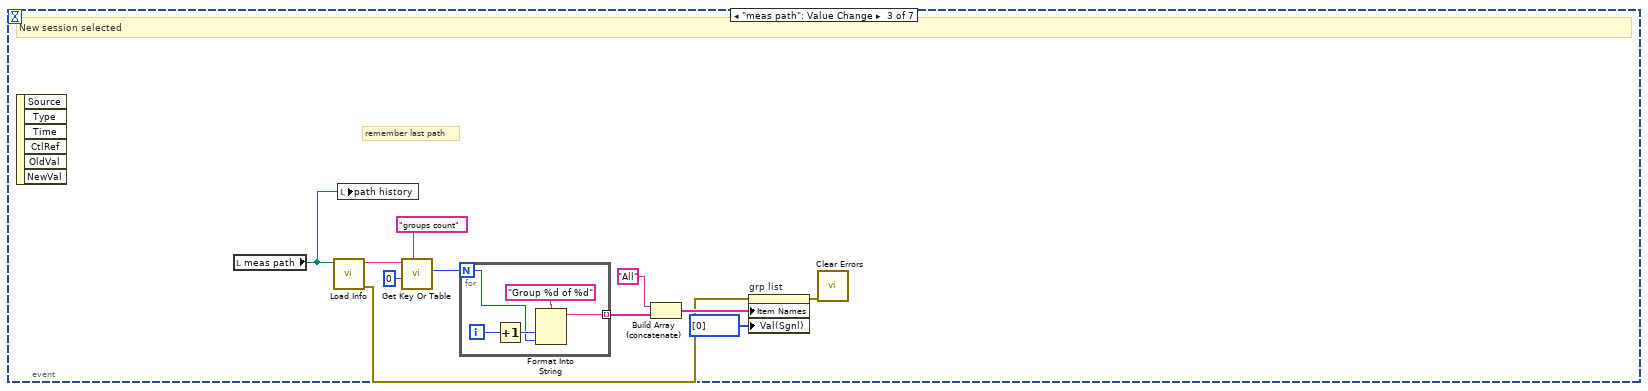
[diagram p4: hidden frame]
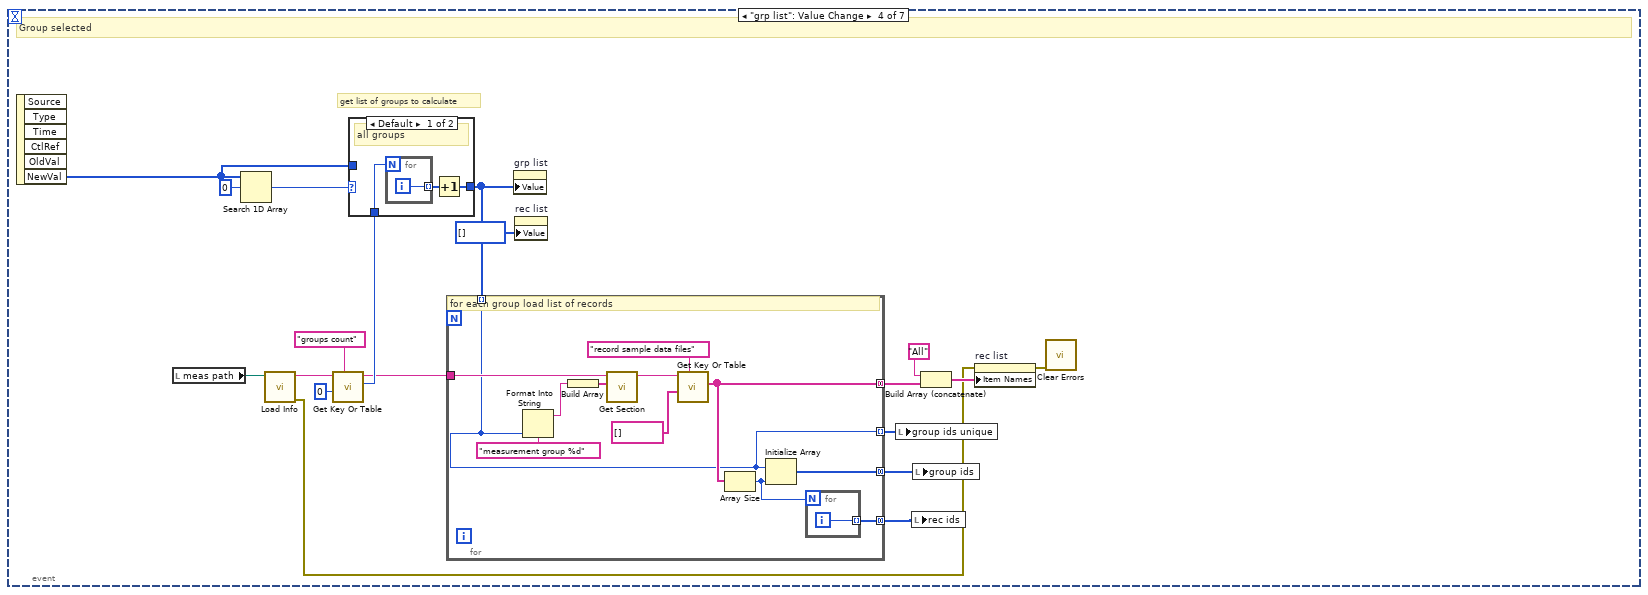
[diagram p5: hidden frame]
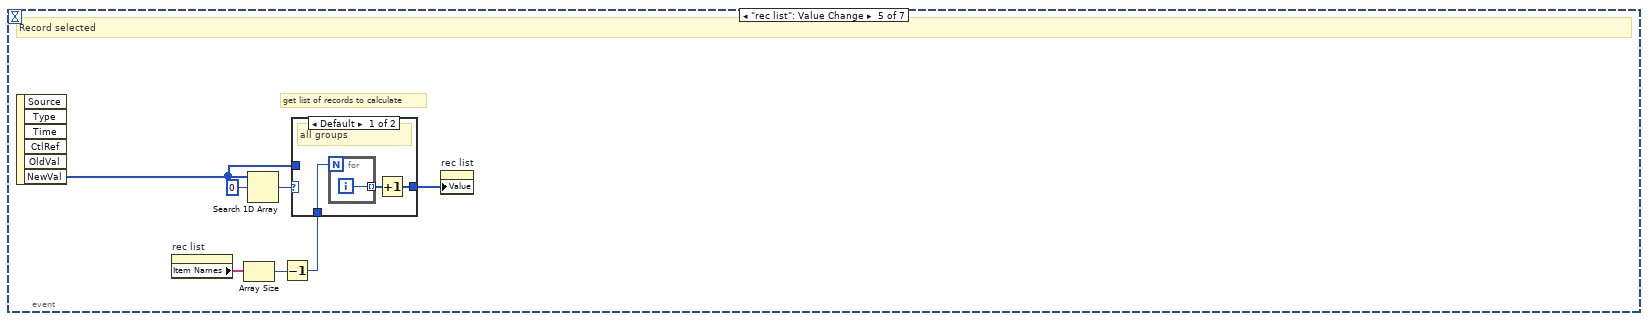
[diagram p7: hidden frame]
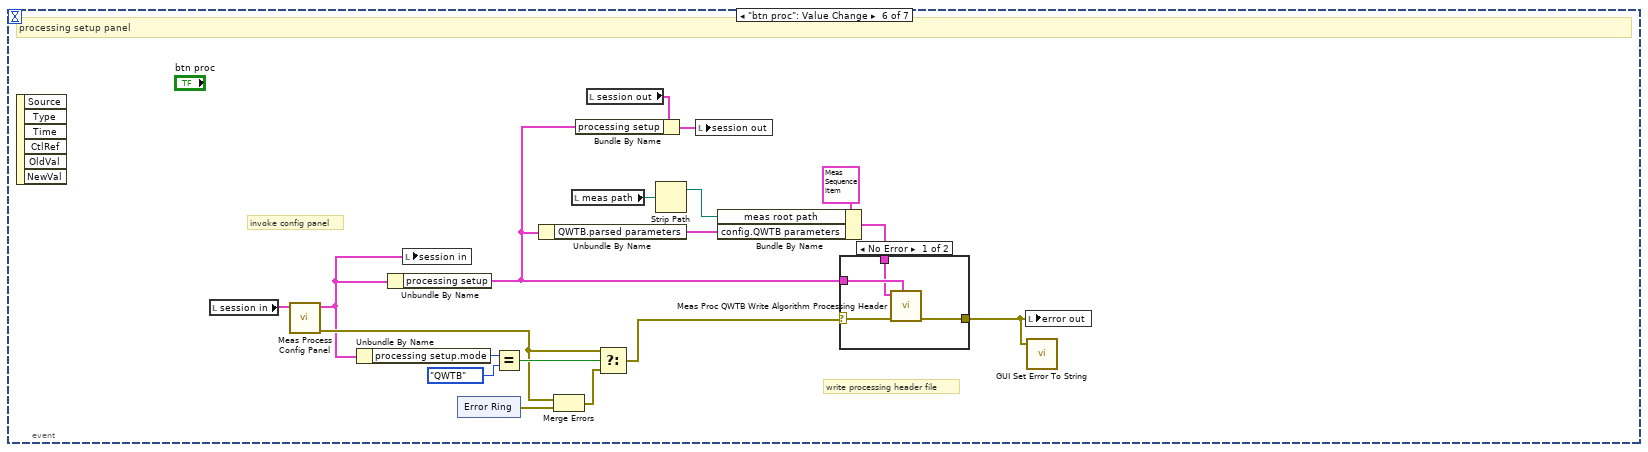
[diagram p9: hidden frame]
diagram:
  w29 = string[] [] ("Item Names")
  # "local variabel - no touchy!"
  # "register panel\ncontrols for SGUI lib"
  n1 = while {
    tunnel: [w31] -> w26
    stop <- w31 stop-if-true
    n2 = event shown="[6] \"btn ok\": Value Change" {
      selector: _ -> [_ _ _ _ _ _ _]
      dyn-events: _ -> [_ _ _ _ _ _ _]
      timeout: _ -> [_ _ _ _ _ _ _]
      tunnel: [_ TRUE _ _ _ _ _] -> w31
      event Timeout {
        n3 = event-data() -> ()  [unwired: 1 in, 3 out]
      }
      event "btn cancel": Value Change; Panel Close {
        n4 = event-data() -> ()  [unwired: 1 in, 3 out]
      }
      event "meas path": Value Change {
        # "remember last path"
        # "New session selected"
        n5 = event-data() -> ()  [unwired: 1 in, 6 out]
        n6 = local read "meas path"() -> (w33:path)
        n7 = call "Load Info.vi"("filename"=w33) -> ("error out"=w37:errorcluster, "info data"=w43:string)  [unwired: 9 in]
        n8 = local write "path history"(w33) -> ()
        n9 = call-poly "Get Key Or Table.vi"("key description"="groups count", "numeric"=i64 0, "info data"=w43) -> ("value"=w41:i64)  [unwired: 5 in, 3 out]
        n10 = for {
          N: w41 -> [w45]
          tunnel: [w44] -> w40 mode=indexing
          i -> [w48]
          n11 = Increment(x=w48) -> (x+1=w47:i32)
          n12 = Format Into String(format string="Group %d of %d", w47, w45) -> (resulting string=w44:string)  [unwired: 2 in, 1 out]
        }
        n13 = Build Array (concatenate)("All", w40) -> (w38:string[])
        n14 = property on="grp list" class="LstBox (strict)"(error in=w37, "Item Names"=w38, "Val(Sgnl)"=i32[] [0] ("Value (Signaling)")) -> (error out=w34:errorcluster)  [unwired: 1 in, 1 out]
        n15 = call <vilib>:"Clear Errors.vi"("error in (no error)"=w34) -> ()  [unwired: 5 in, 2 out]
      }
      event "grp list": Value Change {
        # "get list of groups to calculate"
        # "Group selected"
        n16 = event-data() -> ("NewVal"=w61:i32[])  [unwired: 1 in, 5 out]
        n17 = local read "meas path"() -> (w67:path)
        n18 = Search 1D Array(1D array=w61, element=0) -> (index of element=w62:i32)  [unwired: 1 in]
        n19 = call "Load Info.vi"("filename"=w67) -> ("error out"=w55:errorcluster, "info data"=w66:string)  [unwired: 9 in]
        n20 = call-poly "Get Key Or Table.vi"("key description"="groups count", "numeric"=i64 0, "info data"=w66) -> ("value"=w60:i64, "info data out"=w59:string)  [unwired: 5 in, 2 out]
        n21 = case shown="Default" w62 {
          tunnel: w61 -> [_ w72]
          tunnel: [w68 w72] -> w53
          tunnel: w60 -> [w70 _]
          frame Default {
            # "all groups"
            n22 = for {
              N: w70 -> [_]
              tunnel: [w71] -> w69 mode=indexing
              i -> [w71]
            }
            n23 = Increment(x=w69) -> (x+1=w68:i32[])
          }
          frame -1 {
            # "selected only"
          }
        }
        n24 = for {
          tunnel: w59 -> [w83]
          tunnel: w53 -> [w75] mode=indexing
          tunnel: [w77] -> w58 mode=concatenating
          tunnel: [w76] -> w51 mode=concatenating
          tunnel: [w75] -> w50 mode=indexing
          tunnel: [w73] -> w49 mode=concatenating
          # "for each group load list of records"
          n25 = Format Into String(format string="measurement group %d", w75) -> (resulting string=w82:string)  [unwired: 2 in, 1 out]
          n26 = Build Array(w82) -> (w81:string[])
          n27 = call "Get Section.vi"("sections"=w81, "info data"=w83) -> ("section part"=w80:string)  [unwired: 8 in, 1 out]
          n28 = call-poly "Get Key Or Table.vi"("key description"="record sample data files", "string"=string[] [], "info data"=w80) -> ("value"=w77:string[])  [unwired: 5 in, 3 out]
          n29 = Array Size(array=w77) -> (size(s)=w74:i32)
          n30 = Initialize Array(w75, w74) -> (w76:i32[])
          n31 = for {
            N: w74 -> [_]
            tunnel: [w85] -> w73 mode=indexing
            i -> [w85]
          }
        }
        n32 = property on="grp list" class="LstBox (strict)"("Value"=w53) -> ()  [unwired: 2 in, 2 out]
        n33 = property on="rec list" class="LstBox (strict)"("Value"=i32[] [] ("rec list")) -> ()  [unwired: 2 in, 2 out]
        n34 = local write "group ids unique"(w50) -> ()
        n35 = local write "rec ids"(w49) -> ()
        n36 = local write "group ids"(w51) -> ()
        n37 = Build Array (concatenate)("All", w58) -> (w56:string[])
        n38 = property on="rec list" class="LstBox (strict)"(error in=w55, "Item Names"=w56) -> (error out=w54:errorcluster)  [unwired: 1 in, 1 out]
        n39 = call <vilib>:"Clear Errors.vi"("error in (no error)"=w54) -> ()  [unwired: 5 in, 2 out]
      }
      event "rec list": Value Change {
        # "get list of records to calculate"
        # "Record selected"
        n40 = event-data() -> ("NewVal"=w90:i32[])  [unwired: 1 in, 5 out]
        n41 = property on="rec list" class="LstBox (strict)"() -> ("Item Names"=w89:string[])  [unwired: 2 in, 2 out]
        n42 = Array Size(array=w89) -> (size(s)=w88:i32)
        n43 = Search 1D Array(1D array=w90, element=0) -> (index of element=w91:i32)  [unwired: 1 in]
        n44 = Decrement(x=w88) -> (x-1=w87:i32)
        n45 = case shown="Default" w91 {
          tunnel: w90 -> [_ w97]
          tunnel: [w93 w97] -> w86
          tunnel: w87 -> [w95 _]
          frame Default {
            # "all groups"
            n46 = for {
              N: w95 -> [_]
              tunnel: [w96] -> w94 mode=indexing
              i -> [w96]
            }
            n47 = Increment(x=w94) -> (x+1=w93:i32[])
          }
          frame -1 {
            # "selected only"
          }
        }
        n48 = property on="rec list" class="LstBox (strict)"("Value"=w86) -> ()  [unwired: 2 in, 2 out]
      }
      event "btn proc": Value Change {
        # "write processing header file"
        # "invoke config panel"
        # "processing setup panel"
        n49 = event-data() -> ()  [unwired: 1 in, 6 out]
        n50 = local read "session in"() -> (w115:T1)
        n51 = call "Meas Process Config Panel.vi"("session in"=w115) -> ("error out"=w111:errorcluster, "session out"=w108:T1)  [unwired: 9 in]
        n52 = Unbundle By Name(w108) -> ("processing setup.mode"=w114:T56)
        n53 = Unbundle By Name(w108) -> ("processing setup"=w100:T55)
        n54 = local write "session in"(w108) -> ()
        n55 = xnode "Error Ring"() -> ("error out"=w110:errorcluster)
        n56 = Equal?(x=w114, y=Meas_Process_Mode."QWTB" ("processing setup.mode")) -> (x = y?=w112:bool)
        n57 = Unbundle By Name(w100) -> ("QWTB.parsed parameters"=w104:T50[])
        n58 = Merge Errors(w111, w110) -> (w109:errorcluster)
        n59 = local read "meas path"() -> (w106:path)
        n60 = local read "session out"() -> (w101:T1)
        n61 = Bundle By Name(cluster=w101, "processing setup"=w100) -> (w99:T1)
        n62 = Select(t=w111, s=w112, f=w109) -> (s? t:f=w102:errorcluster)
        n63 = Strip Path(path=w106) -> (stripped path=w105:path)  [unwired: 1 out]
        n64 = local write "session out"(w99) -> ()
        n65 = Bundle By Name(cluster=T44 {"config"={"fs [Hz]"=0.0, "count [smpl]"=0, "aperture [s]"=0.0, "trigger"={"source"=enum."Immediate", "level [V]"=0.0, "coupling"=enum."DC", "slope"=enum."POS"}, "ranges [Vpk]"=[], "QWTB parameters"=[]}, "data file path"=path "", "header file path"=path "", "group id"=0, "average id"=0, "group done?"=FALSE, "adc modified?"=FALSE, "source modified?"=FALSE, "progress [%]"=0.0, "groups cnt"=0, "average cnt"=0, "data file relative path"="", "meas root path"=path "", "calculate?"=FALSE} ("sequence item"), "meas root path"=w105, "config.QWTB parameters"=w104) -> (w103:T44)
        n66 = case shown="No Error" w102 {
          selector: w102 -> [w117 w120]
          tunnel: w100 -> [w119 _]
          tunnel: w103 -> [w118 _]
          tunnel: [w116 w120] -> w98
          frame No Error {
            n67 = call "Meas Proc QWTB Write Algorithm Processing Header.vi"("processing setup"=w119, "error in"=w117, "sequence item"=w118) -> ("error out"=w116:errorcluster)  [unwired: 8 in]
          }
          frame Error {
          }
        }
        n68 = local write "error out"(w98) -> ()
        n69 = call "GUI Set Error To String.vi"("error in (no error)"=w98) -> ()  [unwired: 4 in]
      }
      event "btn ok": Value Change {
        # "Start batch processing"
        n70 = event-data() -> ()  [unwired: 1 in, 6 out]
        n71 = local read "session in"() -> (w130:T1)
        n72 = Unbundle By Name(w130) -> ("processing setup.QWTB.selected alg id"=w129:string)
        n73 = local read "meas path"() -> (w144:path)
        n74 = call "SGUI Set Control Enabled State By Groups.vi"("group name to enable (none)"="qbbusy") -> ("error out"=w134:errorcluster)  [unwired: 9 in, 1 out]
        n75 = Bundle By Name(cluster=T44 {"config"={"fs [Hz]"=0.0, "count [smpl]"=0, "aperture [s]"=0.0, "trigger"={"source"=enum."Immediate", "level [V]"=0.0, "coupling"=enum."DC", "slope"=enum."POS"}, "ranges [Vpk]"=[], "QWTB parameters"=[]}, "data file path"=path "", "header file path"=path "", "group id"=0, "average id"=0, "group done?"=FALSE, "adc modified?"=FALSE, "source modified?"=FALSE, "progress [%]"=0.0, "groups cnt"=0, "average cnt"=0, "data file relative path"="", "meas root path"=path "", "calculate?"=FALSE} ("sequence item"), "header file path"=w144) -> (w142:T44)
        n76 = local read "group ids unique"() -> (w145:i32[])
        n77 = call "SGUI Set Boolean State By Label.vi"("error in"=w134) -> ("error out"=w133:errorcluster)  [unwired: 9 in, 1 out]
        n78 = local read "group ids"() -> (w146:i32[])
        n79 = property on="rec list" class="LstBox (strict)"() -> ("Item Names"=w140:string[], "Value"=w138:i32[])  [unwired: 2 in, 2 out]
        n80 = local read "rec ids"() -> (w141:i32[])
        n81 = Array Size(array=w138) -> (size(s)=w137:i32)
        n82 = for {
          tunnel: w146 -> [w163]
          tunnel: w145 -> [w148] mode=indexing
          tunnel: w142 -> [w166]
          tunnel: w141 -> [w162]
          shift-right: [w151] -> w128
          shift-left: w133 -> [w160]
          tunnel: w140 -> [w159]
          tunnel: w138 -> [w158]
          shift-right: [w156] -> _
          shift-left: 0 -> [w155]
          tunnel: w137 -> [w154]
          tunnel: w129 -> [w149]
          tunnel: [w147] -> w126
          stop <- w150 stop-if-true
          # "for each group of records"
          n83 = Equal?(x=w163, y=w148) -> (x = y?=w164:bool[])
          n84 = for {
            tunnel: w164 -> [w191] mode=indexing
            tunnel: w163 -> [w196] mode=indexing
            tunnel: [w196] -> _ mode=indexing if=w191
            tunnel: [w195] -> w161 mode=indexing if=w191
            tunnel: w162 -> [w195] mode=indexing
            tunnel: w159 -> [w194]
            tunnel: w158 -> [w193] mode=indexing
            tunnel: [w192] -> w157 mode=indexing if=w191
            n85 = Index Array(array=w194, index=w193) -> (element=w192:string)
          }
          n86 = Bundle By Name(cluster=w166, "group id"=w148) -> (w165:T44)
          n87 = for {
            N -> [w175]
            tunnel: w165 -> [w169]
            tunnel: w161 -> [w189] mode=indexing
            shift-right: [w173] -> w152
            shift-left: w160 -> [w186]
            tunnel: w157 -> [w184] mode=indexing
            shift-right: [w182] -> w156
            shift-left: w155 -> [w183]
            tunnel: w154 -> [w181]
            tunnel: w149 -> [w168]
            tunnel: [w167] -> w147
            i -> [w177]
            stop <- w172 stop-if-true
            # "for each record in the group"
            n88 = Increment(x=w177) -> (x+1=w176:i32)
            n89 = Equal?(x=w175, y=w176) -> (x = y?=w174:bool)
            n90 = Increment(x=w189) -> (x+1=w180:i32)
            n91 = Increment(x=w183) -> (x+1=w182:i32)
            n92 = Bundle By Name(cluster=w169, "average id"=w180, "group done?"=w174) -> (w167:T44)
            n93 = Format Into String(format string="<tc=gold><b>Processing record: <tc=cyan>%s</tc>\nAlgorithm: <tc=cyan>%s</tc>\n<tc=gold><b>Progress: %d of %d ...", error in=w186, w184, w168, w182, w181) -> (resulting string=w178:string, error out=w187:errorcluster)  [unwired: 1 in]
            n94 = call-poly "SGUI Assign String With Tags.vi"("error in"=w187, "label(s) (empty)"="status" ("string (empty)"), "string (empty)"=w178) -> ("error out"=w188:errorcluster)  [unwired: 7 in, 1 out]
            n95 = local read "session in"() -> (w190:T1)
            n96 = call "Meas Process Record.vi"("session"=w190, "error in"=w188, "sequence item"=w167) -> ("error out"=w170:errorcluster)  [unwired: 8 in]
            n97 = call "SGUI Get Boolean State By Label.vi"("error in"=w170) -> ("error out"=w173:errorcluster, "binary state out"=w171:bool)  [unwired: 8 in, 1 out]
            n98 = Compound Arithmetic op=OR(w171, w170) -> (w172:bool)
          }
          n99 = call "SGUI Get Boolean State By Label.vi"("error in"=w152) -> ("error out"=w151:errorcluster, "binary state out"=w153:bool)  [unwired: 8 in, 1 out]
          n100 = Compound Arithmetic op=OR(w153, w152) -> (w150:bool)
        }
        n101 = call "GUI FFT Update.vi"("error in"=w128, "sequence item"=w126) -> ("error out"=w127:errorcluster)  [unwired: 9 in]
        n102 = call "SGUI Set Control Enabled State By Groups.vi"("error in"=w127, "group name to enable (none)"="qbready") -> ("error out"=w132:errorcluster)  [unwired: 8 in, 1 out]
        n103 = call "SGUI Set Boolean State By Label.vi"("error in"=w132) -> ("error out"=w131:errorcluster)  [unwired: 9 in, 1 out]
        n104 = local write "error out"(w131) -> ()
        n105 = call "GUI Set Error To String.vi"("error in (no error)"=w131) -> ()  [unwired: 4 in]
      }
    }
  }
  n106 = control-ref of="btn stop"() -> (w14:refnum<vi>)
  n107 = control-ref of="btn ok"() -> (w15:refnum<vi>)
  n108 = control-ref of="btn cancel"() -> (w13:refnum<vi>)
  n109 = control-ref of="btn proc"() -> (w12:refnum<vi>)
  n110 = control-ref of="grp list"() -> (w11:refnum<vi>)
  n111 = control-ref of="rec list"() -> (w10:refnum<vi>)
  n112 = call "SGUI Register Controls.vi"("error in"="error in", "register mode (overwrite)"=SGUI_Assign_References_Mode."Add to stack") -> ("assigned ID"=w2:string, "error out"=w22:errorcluster)  [unwired: 15 in, 1 out]
  n113 = property on="meas path" class="Path"("StartPath"="path history", "Value"=path "" ("meas path")) -> ()  [unwired: 2 in, 2 out]
  n114 = Build Array(w15, w13, w12, w11, w10) -> (w19:refnum<vi>[])
  n115 = Build Array(w14) -> (w18:refnum<vi>[])
  n116 = Bundle(w19) -> (w16:cluster{refnum<vi>[]})  [unwired: 1 in]
  n117 = Bundle(w18) -> (w17:cluster{refnum<vi>[]})  [unwired: 1 in]
  n118 = Build Array(w16, w17) -> (w20:cluster{refnum<vi>[]}[])
  n119 = call "SGUI Register Controls Groups.vi"("control groups"=w20, "error in"=w22, "groups names"="qbready\nqbbusy", "register mode (overwrite)"=SGUI_Assign_References_Mode."Add to stack") -> ("assigned ID"=w1:string, "error out"=w9:errorcluster)  [unwired: 14 in]
  n120 = call "SGUI Set Control Enabled State By Groups.vi"("error in"=w9, "group name to enable (none)"="qbready") -> ("error out"=w7:errorcluster)  [unwired: 8 in, 1 out]
  n121 = call "SGUI Set Boolean State By Label.vi"("error in"=w7) -> ("error out"=w6:errorcluster)  [unwired: 9 in, 1 out]
  n122 = property on="grp list" class="LstBox (strict)"("Item Names"=w29) -> ()  [unwired: 2 in, 2 out]
  n123 = property on="rec list" class="LstBox (strict)"("Item Names"=w29) -> ()  [unwired: 2 in, 2 out]
  n124 = call-poly "SGUI Assign String With Tags.vi"("error in"=w6, "label(s) (empty)"="status", "string (empty)"="<bc=black><tc=gold><b>Select measurement session") -> ("error out"=→"error out":errorcluster)  [unwired: 7 in, 1 out]
  n125 = flat-sequence {
    tunnel: w26 -> [_]
    tunnel: w2 -> [w198]
    tunnel: w1 -> [w197]
    frame #0 {
      w199 = SGUI_Assign_References_Mode."Release ID" ("register mode (overwrite)")
      # "on exit action - release GUI controls"
      n126 = call "SGUI Register Controls Groups.vi"("register mode (overwrite)"=w199, "controls ID (empty)"=w197) -> ("error out"=w200:errorcluster)  [unwired: 16 in, 1 out]
      n127 = call "SGUI Register Controls.vi"("error in"=w200, "register mode (overwrite)"=w199, "controls ID (empty)"=w198) -> ("error out"=w201:errorcluster)  [unwired: 14 in, 2 out]
      n128 = call <vilib>:"Clear Errors.vi"("error in (no error)"=w201) -> ()  [unwired: 5 in, 2 out]
    }
  }
  "session out" <- "session in"
